vi "ApplicationConfigurationName --constant.vi"() -> (2 "AppConfigName":string, 3 "AppName":string)   [LabVIEW 2021, in "IApplicationConfiguration.lvclass"]
uses:
  IApplicationConfiguration.lvclass
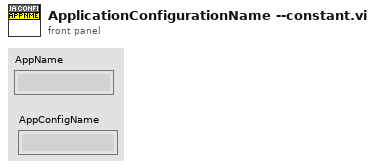
[diagram p1: front panel]
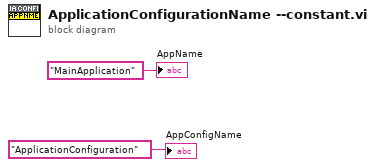
[diagram p0: block diagram]
diagram:
  "AppConfigName" <- "ApplicationConfiguration" ("AppConfigName")
  "AppName" <- "MainApplication" ("AppName")
